vi "configure.vi"(8 "error in (no error)":errorcluster, 11 "GenericPlugin in":refnum<class "StimulatorDL090503.lvclass">) -> (0 "error out":errorcluster, 3 "GenericPlugin out":refnum<class "StimulatorDL090503.lvclass">)   [LabVIEW 2010, in "StimulatorDL090503.lvclass"]
doc: "The dynamic dispatch version of this VI loads and displays the configuration file associated with the plug-in object. The user modify and save the configuration data."
uses:
  StimulatorDL090503.lvclass
  common/xcontrols/XComponentSpecification/XComponentSpecification/XComponentSpecification.xctl
  StimulatorDL090503.lvclass/StimulatorDL090503.ctl
  SignalWriter/GenericSignalWriter/GenericSignalWriter/GenericSignalWriter.lvclass
  common/classes/GenericComponent/GenericComponent/GenericComponent.lvclass
panel:
  in  "signalWriter spec":T1(xcontrol)
  in  "save button":bool
  in  "cancel button":bool
  in  "Sampling rate":dbl[unit]
  out "Configuration":string
  # "Configure StimulatorDL090503"
  # "SignalWriter"
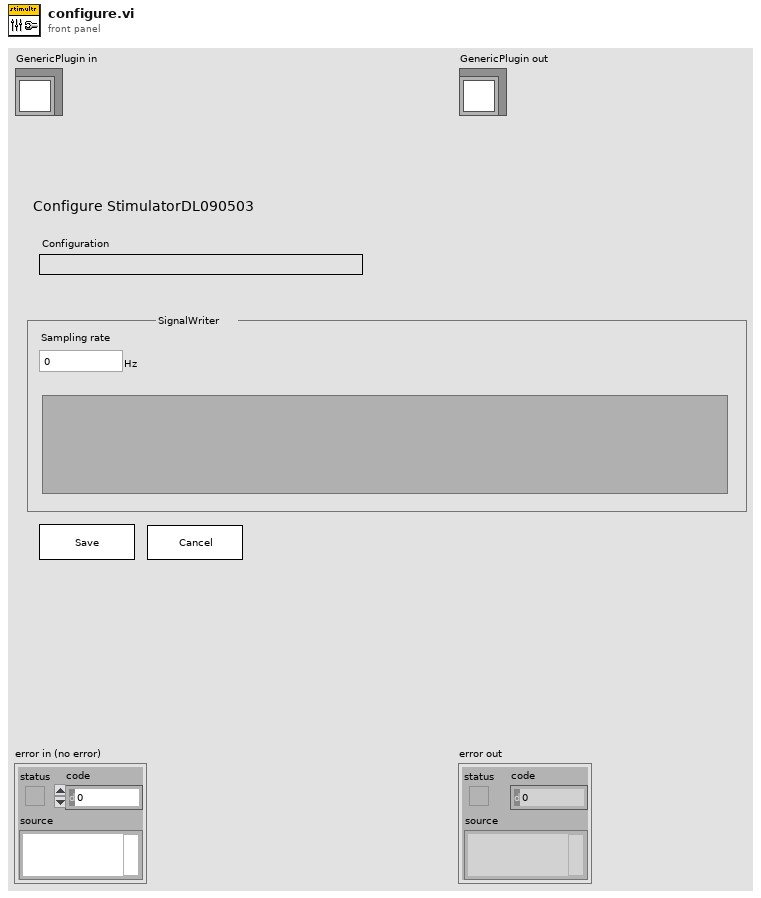
[diagram p1: front panel]
types:
  T1 = cluster{"class path":string, "configuration":string, "label":string, "settings name":string}
  T2 = typedef "plugin_specification.ctl" = cluster{"class path":string, "configuration":string, "label":string, "settings name":string}
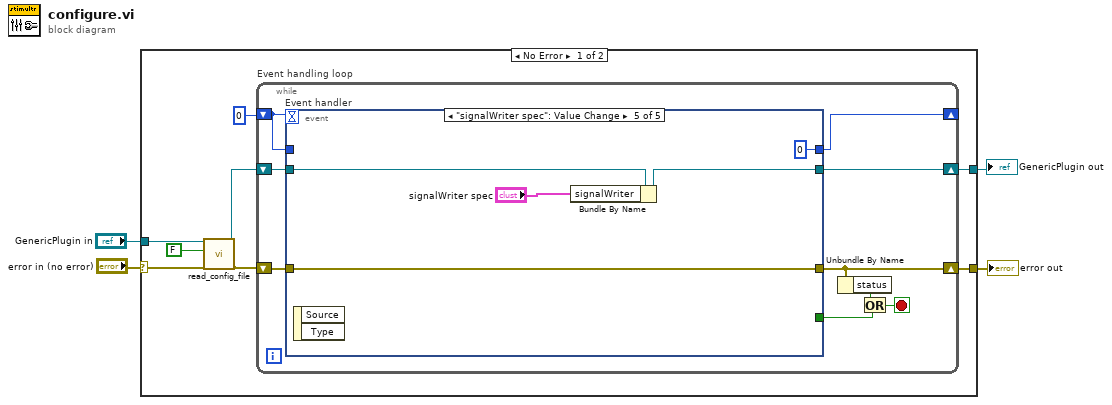
[diagram p0: block diagram]
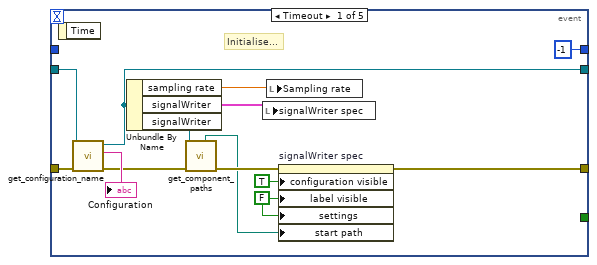
[diagram p2: hidden frame]
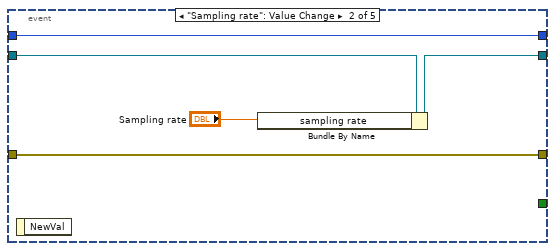
[diagram p3: hidden frame]
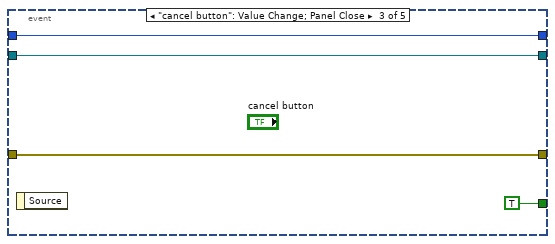
[diagram p4: hidden frame]
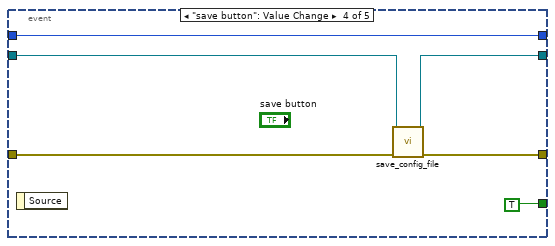
[diagram p5: hidden frame]
diagram:
  n1 = case shown="No Error" "error in (no error)" {
    selector: "error in (no error)" -> [w8 w57]
    tunnel: [w12 w57] -> w2
    tunnel: "GenericPlugin in" -> [w6 w56]
    tunnel: [w10 w56] -> w1
    frame No Error {
      n2 = call-dynamic "read_config_file.vi"("error in (no error)"=w8, "force load?"=FALSE, "GenericPlugin in"=w6) -> ("error out"=w7:errorcluster, "GenericPlugin out"=w5:refnum<class "StimulatorDL090503.lvclass">)  [unwired: 7 out]
      n3 = while "Event handling loop" {
        shift-right: [w16] -> w12
        shift-left: w7 -> [w21]
        shift-right: [w19] -> _
        shift-left: 0 -> [w20]
        shift-right: [w17] -> w10
        shift-left: w5 -> [w18]
        stop <- w13 stop-if-true
        n4 = event "Event handler" shown="[4] \"signalWriter spec\": Value Change" {
          selector: _ -> [_ _ _ _ _]
          dyn-events: _ -> [_ _ _ _ _]
          timeout: w20 -> [_ _ _ _ _]
          tunnel: w21 -> [w33 w40 w44 w48 w51]
          tunnel: [w26 w40 w44 w46 w51] -> w16
          tunnel: w20 -> [_ w39 w43 w50 _]
          tunnel: [-1 w39 w43 w50 0] -> w19
          tunnel: [_ _ TRUE TRUE _] -> w14
          tunnel: w18 -> [w31 w38 w41 w45 w55]
          tunnel: [w29 w37 w41 w47 w54] -> w17
          event Timeout {
            w22 = FALSE ("label visible")
            # "Initialise..."
            n5 = event-data() -> ()  [unwired: 2 out]
            n6 = call "get_configuration_name.vi"("error in (no error)"=w33, "GenericPlugin.lvclass in"=w31) -> ("error out"=w30:errorcluster, "configuration name"=→"Configuration":string, "GenericPlugin.lvclass out"=w29:refnum<class "StimulatorDL090503.lvclass">)  [unwired: 7 in]
            n7 = Unbundle By Name(w29) -> ("sampling rate"=w34:dbl[unit], "signalWriter"=w25:T2, "signalWriter"=w28:refnum<class "GenericSignalWriter.lvclass">)
            n8 = call-dynamic "get_component_paths.vi"("error in (no error)"=w30, "GenericComponent in"=w28) -> ("error out"=w27:errorcluster, "component type directory"=w24:path)  [unwired: 4 in, 4 out]
            n9 = local write "signalWriter spec"(w25) -> ()
            n10 = local write "Sampling rate"(w34) -> ()
            n11 = property on="signalWriter spec" class="XComponentSpecification (strict"(error in=w27, "configuration visible"=TRUE, "label visible"=w22, "settings"=w22, "start path"=w24) -> (error out=w26:errorcluster)  [unwired: 1 in, 1 out]
          }
          event "Sampling rate": Value Change {
            n12 = event-data() -> ()  [unwired: 2 out]
            n13 = Bundle By Name(cluster=w38, "sampling rate"="Sampling rate") -> (w37:refnum<class "StimulatorDL090503.lvclass">)
          }
          event "cancel button": Value Change; Panel Close {
            n14 = event-data() -> ()  [unwired: 2 out]
          }
          event "save button": Value Change {
            n15 = event-data() -> ()  [unwired: 2 out]
            n16 = call-dynamic "save_config_file.vi"("error in (no error)"=w48, "GenericPlugin in"=w45) -> ("error out"=w46:errorcluster, "GenericPlugin out"=w47:refnum<class "StimulatorDL090503.lvclass">)  [unwired: 1 in, 7 out]
          }
          event "signalWriter spec": Value Change {
            n17 = event-data() -> ()  [unwired: 3 out]
            n18 = Bundle By Name(cluster=w55, "signalWriter"="signalWriter spec") -> (w54:refnum<class "StimulatorDL090503.lvclass">)
          }
        }
        n19 = Unbundle By Name(w16) -> ("status"=w15:bool)
        n20 = Or(x=w15, y=w14) -> (x .or. y?=w13:bool)
      }
    }
    frame Error {
    }
  }
  "error out" <- w2
  "GenericPlugin out" <- w1
